vi "Timestamp to ISO8601 Day.vi"(9 "UTC? (F)":bool, 11 "Timestamp (now)":timestamp) -> (1 "Day of Year":i32, 2 "ISO Weekday":i32, 3 "ISO Day":T1)   [LabVIEW 2013]
doc: "- ISO Day is an enum starting on Monday (first day of ISO week)\n\n- ISO Weekday is a 1-based numeral that is helpful for ISO standard calculations (1: Monday, 2: Tuesday, ..., 7: Sunday)\n\n- Day of year is also a 1-based numeral where January 1st is 001. This series ends at 365 or 366 days, depending on leap years."
uses:
  ISO Day -- enum.ctl
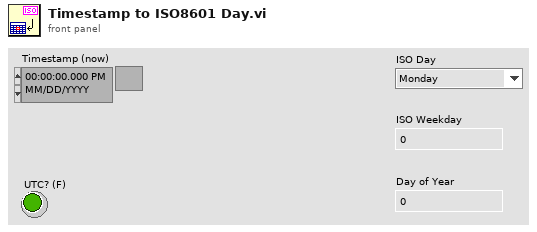
[diagram p1: front panel]
types:
  T1 = typedef "ISO Day -- enum.ctl" = enum16{"Monday", "Tuesday", "Wednesday", "Thursday", "Friday", "Saturday", "Sunday"}
  T2 = typedef "LVDateTimeRec.ctl" = cluster{"fractional second":dbl, "second":i32, "minute":i32, "hour":i32, "day of month":i32, "month":i32, "year":i32, "day of week":i32, "day of year":i32, "DST":i32}
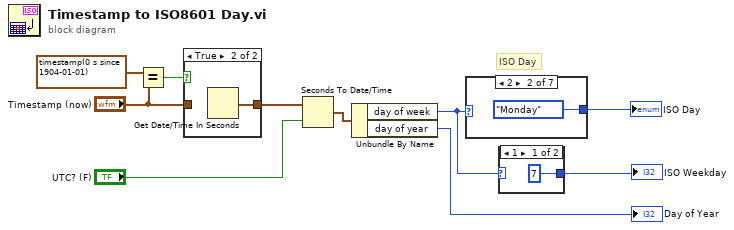
[diagram p0: block diagram]
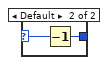
[diagram p2: hidden frame]
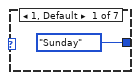
[diagram p3: hidden frame]
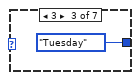
[diagram p4: hidden frame]
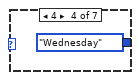
[diagram p5: hidden frame]
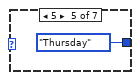
[diagram p6: hidden frame]
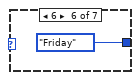
[diagram p7: hidden frame]
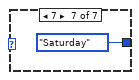
[diagram p8: hidden frame]
diagram:
  # "ISO Day"
  n1 = Equal?(x=timestamp(0 s since 1904-01-01), y="Timestamp (now)") -> (x = y?=w9:bool)
  n2 = case shown="True" w9 {
    tunnel: [w11 w12] -> w7
    tunnel: "Timestamp (now)" -> [w11 _]
    frame False {
    }
    frame True {
      n3 = Get Date/Time In Seconds() -> (seconds since 1Jan1904=w12:timestamp)
    }
  }
  n4 = Seconds To Date/Time(time stamp (now)=w7, to UTC (F)="UTC? (F)") -> (date time rec=w5:T2)
  n5 = Unbundle By Name(w5) -> ("day of week"=w3:i32, "day of year"=→"Day of Year":i32)
  n6 = case shown="2" w3 {
    tunnel: [ISO_Day_--_enum."Sunday" ("Day of Week") ISO_Day_--_enum."Monday" ("Day of Week") ISO_Day_--_enum."Tuesday" ("Day of Week") ISO_Day_--_enum."Wednesday" ("Day of Week") ISO_Day_--_enum."Thursday" ("Day of Week") ISO_Day_--_enum."Friday" ("Day of Week") ISO_Day_--_enum."Saturday" ("Day of Week")] -> w6
    frame 1, Default {
    }
    frame 2 {
    }
    frame 3 {
    }
    frame 4 {
    }
    frame 5 {
    }
    frame 6 {
    }
    frame 7 {
    }
  }
  "ISO Day" <- w6
  n7 = case shown="1" w3 {
    selector: w3 -> [_ w22]
    tunnel: [7 w21] -> w2
    frame 1 {
    }
    frame Default {
      n8 = Decrement(x=w22) -> (x-1=w21:i32)
    }
  }
  "ISO Weekday" <- w2
